vi "TopTemperatureMeasure.vi"() -> ()   [LabVIEW 2016]
uses:
  type def/ZAddress.ctl
  type def/Database.ctl
  TemperatureMeasure/Thermal_type.vi
  user/GrobaLimitVoltage.vi
panel:
  in  "Min.Depth":bool=TRUE
  in  "Max.PRF":bool
  in  "System \nSelection":enum32{"Common", "Frosk", "Griffin", "K2"}(radio)
  in  "Debug":bool
  out "Type Transducer":string="Phase"
  out "PID ON":bool=TRUE
  in  "확인 버튼":bool
  in  "Measured Time for SA":enum32{"5min", "30min"}(radio)=enum."30min"
  in  "Measured\n   Time for volt":enum32{"5min", "30min"}(radio)=enum."30min"
  in  "measSetId(SA modeling)\n(For Temp_Coefficient)":string="29, 37, 44"
  in  "VISA resource":refnum<visa-resource-name>="COM1"
  in  "Thermometer Type":u16(ring)=1 items=["HH506R", "HH506RA"]
  out "CW 2":bool
  in  "S/N(System, Transducer) & S/W":string="PP5327, 22300023, 0.20.17"
  in  "Logfile name":string="log_030905_11_57.txt"
  in  "Database input(hidden)":T1={"DB name"="eagle", "UID"="sel02776", "password"="9ol.(OL>"}
  in  "Boolean":bool
  out "Database":T1={"DB name"="eagle", "UID"="sel02776", "password"="9ol.(OL>"}
  in  "Quit":bool
  in  "Log folder":path=path "C:/temp log data"
  in  "Z Address":T2={"Address"="192.168.52.1", "Port"=1023}
  in  "measSetId(Voltage)\n(For Tempstring)":string="29, 37, 44"
  # "TTS program ver4.0"
  # "Software Version: ver4.0(0001)"
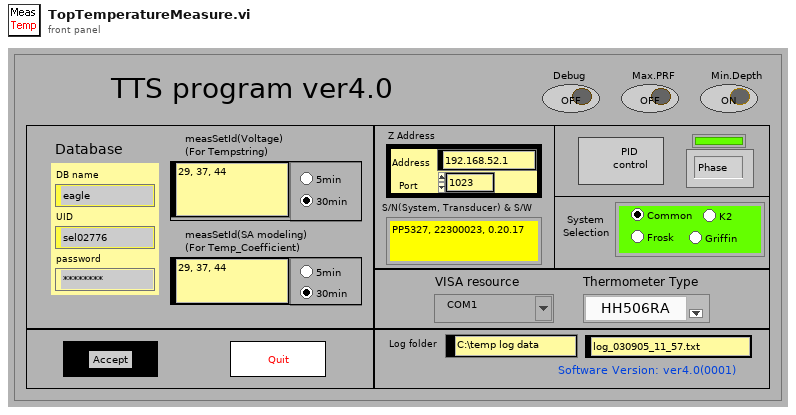
[diagram p1: front panel]
types:
  T1 = typedef "Database.ctl" = cluster{"DB name":string, "UID":string, "password":string}
  T2 = typedef "ZAddress.ctl" = cluster{"Address":string, "Port":u16}
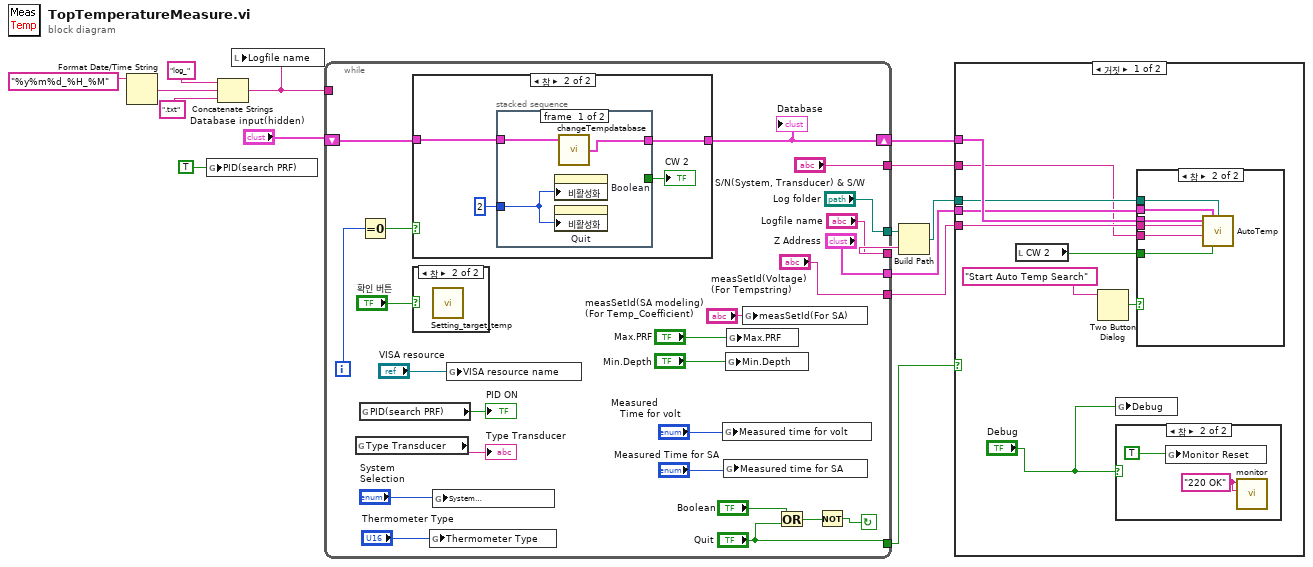
[diagram p0: block diagram]
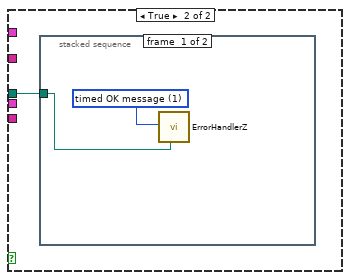
[diagram p4: hidden frame]
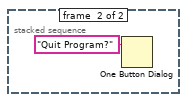
[diagram p5: hidden frame]
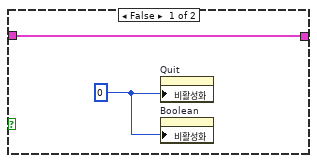
[diagram p7: hidden frame]
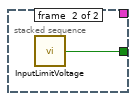
[diagram p8: hidden frame]
diagram:
  n1 = Format Date/Time String(time format string (%c)="%y%m%d_%H_%M") -> (date/time string=w12:string)  [unwired: 2 in]
  n2 = global write "Thermal_type.vi" "PID(search PRF)"(TRUE ("PID ON")) -> ()
  n3 = Concatenate Strings("log_" ("Substring"), w12, ".txt" ("Substring")) -> (w11:string)
  n4 = local write "Logfile name"(w11) -> ()
  n5 = while {
    tunnel: ["Logfile name"] -> w8
    tunnel: ["measSetId(Voltage)\n(For Tempstring)"] -> w6
    tunnel: ["Z Address"] -> w7
    tunnel: ["Log folder"] -> w9
    tunnel: ["Quit"] -> w3
    shift-left: "Database input(hidden)" -> [w36]
    shift-right: [w32] -> w4
    tunnel: w11 -> [_]
    tunnel: ["S/N(System, Transducer) & S/W"] -> w2
    i -> [w38]
    stop <- w39 continue-if-true
    n6 = global read "Thermal_type.vi" "Type Transducer"() -> (→"Type Transducer":string)
    n7 = Equal To 0?(x=w38) -> (x = 0?=w37:bool)
    n8 = global read "Thermal_type.vi" "PID(search PRF)"() -> (→"PID ON":bool)
    n9 = case shown="참" w37 {
      tunnel: [w41 w45] -> w32
      tunnel: w36 -> [w41 w44]
      frame False {
        w40 = 0
        n10 = property on="Quit" class="Bool"("비활성화"=w40) -> ()  [unwired: 2 in, 2 out]
        n11 = property on="Boolean" class="Bool"("비활성화"=w40) -> ()  [unwired: 2 in, 2 out]
      }
      frame True {
        n12 = stacked-sequence {
          tunnel: [w48 _] -> w45
          tunnel: w44 -> [w47 _]
          tunnel: u8 2 ("Write Attribute") -> [w46 _]
          tunnel: [_ w49] -> w42
          frame #0 {
            n13 = property on="Boolean" class="Bool"("비활성화"=w46) -> ()  [unwired: 2 in, 2 out]
            n14 = property on="Quit" class="Bool"("비활성화"=w46) -> ()  [unwired: 2 in, 2 out]
            n15 = call "changeTempdatabase.vi"("Database input(hidden)"=w47) -> ("Database out"=w48:T1)  [unwired: 2 in]
          }
          frame #1 {
            n16 = call "InputLimitVoltage.vi"() -> ("CW 2"=w49:bool)  [unwired: 5 in, 1 out]
          }
        }
        "CW 2" <- w42
      }
    }
    "Database" <- w32
    n17 = case shown="참" "확인 버튼" {
      frame False {
      }
      frame True {
        n18 = call "Setting_target_temp.vi"() -> ()  [unwired: 4 in]
      }
    }
    n19 = global write "Thermal_type.vi" "Thermometer Type"("Thermometer Type") -> ()
    n20 = global write "Thermal_type.vi" "System \nSelection"("System \nSelection") -> ()
    n21 = global write "Thermal_type.vi" "VISA resource name"("VISA resource") -> ()
    n22 = global write "Thermal_type.vi" "Measured time for volt"("Measured\n   Time for volt") -> ()
    n23 = global write "Thermal_type.vi" "Measured time for SA"("Measured Time for SA") -> ()
    n24 = global write "Thermal_type.vi" "Min.Depth"("Min.Depth") -> ()
    n25 = global write "Thermal_type.vi" "Max.PRF"("Max.PRF") -> ()
    n26 = global write "Thermal_type.vi" "measSetId(For SA)"("measSetId(SA modeling)\n(For Temp_Coefficient)") -> ()
    n27 = Or(x="Boolean", y="Quit") -> (x .or. y?=w35:bool)
    n28 = Not(x=w35) -> (.not. x?=w39:bool)
  }
  n29 = Build Path(base path=w9, name or relative path=w8) -> (appended path=w5:path)
  n30 = case shown="거짓" w3 {
    tunnel: w4 -> [w56 _]
    tunnel: w5 -> [w55 w67]
    tunnel: w7 -> [w54 _]
    tunnel: w6 -> [w53 _]
    tunnel: w2 -> [w52 _]
    frame False {
      n31 = local read "CW 2"() -> (w51:bool)
      n32 = Two Button Dialog(message="Start Auto Temp Search") -> (T button?=w57:bool)  [unwired: 2 in]
      n33 = global write "GrobaLimitVoltage.vi" "Debug"("Debug") -> ()
      n34 = case shown="참" "Debug" {
        frame False {
        }
        frame True {
          w59 = "220 OK" ("Received text 2")
          n35 = global write "GrobaLimitVoltage.vi" "Monitor Reset"(TRUE ("Monitor Reset")) -> ()
          n36 = call "monitor.vi"("Received text 4"=w59, "Received text 2"=w59) -> ()  [unwired: 4 in]
        }
      }
      n37 = case shown="참" w57 {
        tunnel: w56 -> [_ w66]
        tunnel: w54 -> [_ w65]
        tunnel: w55 -> [_ w64]
        tunnel: w53 -> [_ w63]
        tunnel: w52 -> [_ w62]
        tunnel: w51 -> [_ w61]
        frame False {
        }
        frame True {
          n38 = call "AutoTemp.vi"("Database"=w66, "Z Address"=w65, "Log file"=w64, "measSetId list"=w63, "Comment(SN)"=w62, "CW"=w61) -> ()  [unwired: 8 in, 2 out]
        }
      }
    }
    frame True {
      n39 = stacked-sequence {
        tunnel: w67 -> [w68 _]
        frame #0 {
          w69 = u16 1 items=["no dialog", "timed OK message", "timed options message"] ("type of dialog (timed opt:2)")
          n40 = call "ErrorHandlerZ.vi"("type of dialog (timed opt:2)"=w69, "Log file"=w68) -> ()  [unwired: 12 in, 6 out]
        }
        frame #1 {
          n41 = One Button Dialog(message="Quit Program?") -> ()  [unwired: 1 in, 1 out]
        }
      }
    }
  }
